vi "Run Action.vi"(8 "Error In":errorcluster, 9 "Timeout (s)":dbl, 10 "Action":string, 11 "Logger In":refnum<class "LoggerAPI.lvclass">) -> (0 "Error Out":errorcluster, 1 "Timeout?":bool, 3 "Logger Out":refnum<class "LoggerAPI.lvclass">)   [LabVIEW 2020, in "LoggerAPI.lvclass"]
uses:
  LoggerAPI.lvclass
  IAction/IAction.lvclass
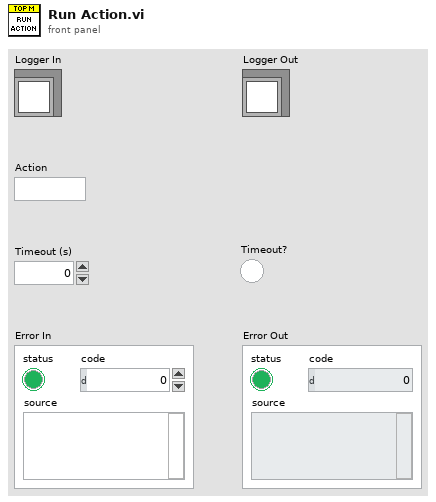
[diagram p1: front panel]
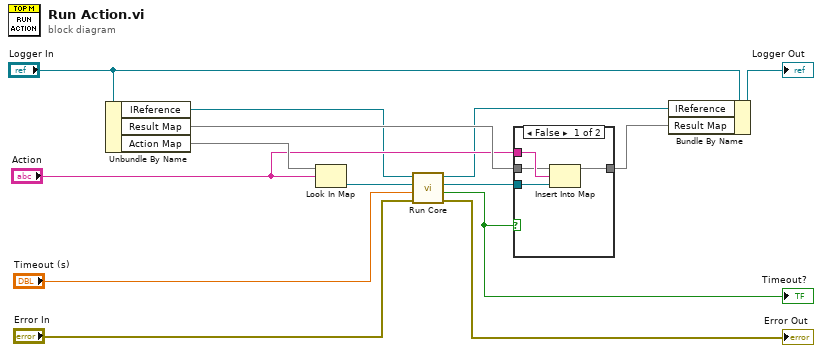
[diagram p0: block diagram]
diagram:
  n1 = Unbundle By Name("Logger In") -> ("IReference"=w8:refnum<class "ILogger.lvclass">, "Result Map"=w11:map{string, refnum<class "IResult.lvclass">}, "Action Map"=w12:map{string, refnum<class "IAction.lvclass">})
  n2 = Look In Map(map=w12, key="Action") -> (value=w6:refnum<class "IAction.lvclass">)  [unwired: 1 in, 1 out]
  n3 = call-dynamic "Run Core.vi"("Error In"="Error In", "Timeout (s)"="Timeout (s)", "Meas In"=w6, "Hardware In"=w8) -> ("Error Out"=→"Error Out":errorcluster, "Timeout?"=w1:bool, "Result Out"=w5:refnum<class "IResult.lvclass">, "Hardware Out"=w7:refnum<class "ILogger.lvclass">)  [unwired: 4 in]
  "Timeout?" <- w1
  n4 = case shown="False" w1 {
    tunnel: "Action" -> [w18 _]
    tunnel: w11 -> [w17 w19]
    tunnel: [w16 w19] -> w10
    tunnel: w5 -> [w15 _]
    frame False {
      n5 = Insert Into Map(map in=w17, key=w18, value=w15) -> (map out=w16:map{string, refnum<class "IResult.lvclass">})  [unwired: 2 out]
    }
    frame True {
    }
  }
  n6 = Bundle By Name(cluster="Logger In", "IReference"=w7, "Result Map"=w10) -> (→"Logger Out":refnum<class "LoggerAPI.lvclass">)
